vi "uA_daq_Check_wearables_profile.vi"(9 "VDUT":string, 10 "Profile":enum16{"SAM", "DIANA", "Other..."}(ring)=enum."Other...", 11 "DUT Voltage Selector":enum16{"3.8VDC", "2.9VDC", "3.7VDC", "4.0VDC"}(ring)) -> (2 "Profile":bool, 3 "Mess":string)   [LabVIEW 2017]
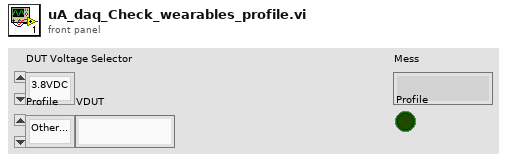
[diagram p1: front panel]
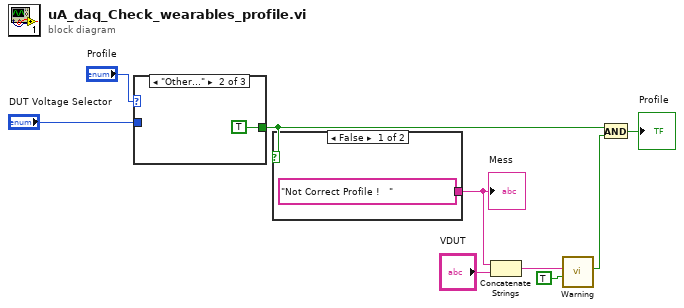
[diagram p0: block diagram]
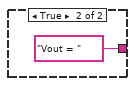
[diagram p2: hidden frame]
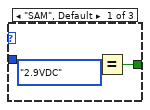
[diagram p3: hidden frame]
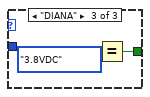
[diagram p4: hidden frame]
diagram:
  n1 = case shown="\"Other...\"" "Profile" {
    tunnel: "DUT Voltage Selector" -> [w11 _ w15]
    tunnel: [w10 TRUE w14] -> w5
    frame "SAM", Default {
      n2 = Equal?(x=w11, y=enum16{"3.8VDC", "2.9VDC", "3.7VDC", "4.0VDC"}."2.9VDC" ("DUT Voltage Selector")) -> (x = y?=w10:bool)
    }
    frame "Other..." {
    }
    frame "DIANA" {
      n3 = Equal?(x=w15, y=enum16{"3.8VDC", "2.9VDC", "3.7VDC", "4.0VDC"}."3.8VDC" ("DUT Voltage Selector")) -> (x = y?=w14:bool)
    }
  }
  n4 = case shown="False" w5 {
    tunnel: ["Not Correct Profile !   " "Vout = "] -> w3
    frame False {
    }
    frame True {
    }
  }
  "Mess" <- w3
  n5 = Concatenate Strings(w3, "VDUT") -> (w1:string)
  n6 = call "Warning"("Enable"=TRUE, "Message"=w1) -> ("OK"=w6:bool)  [unwired: 8 in, 1 out]
  n7 = And(x=w5, y=w6) -> (x .and. y?=→"Profile":bool)
